vi "Disconnect from Slave.vi"(8 "error in (no error)":errorcluster, 11 "ELAN master in":refnum<class "ELAN Master.lvclass">) -> (0 "error out":errorcluster, 3 "ELAN master out":refnum<class "ELAN Master.lvclass">)   [LabVIEW 2021, in "ELAN Master.lvclass"]
doc: "This provides an interface for the master to open a connection to the slave."
uses:
  ELAN Master.lvclass
  ELAN Master.lvclass/ELAN Master.ctl
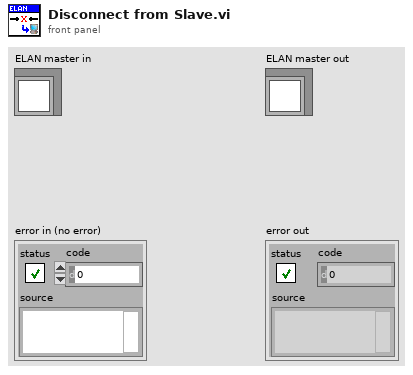
[diagram p1: front panel]
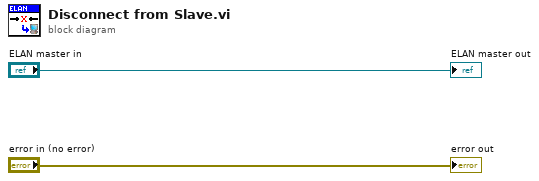
[diagram p0: block diagram]
diagram:
  "error out" <- "error in (no error)"
  "ELAN master out" <- "ELAN master in"
